vi "Projectile_Range.vi"() -> ()   [LabVIEW 2022 SP3]
panel:
  out "Max Height (m)":dbl
  out "Max Range (m)":dbl
  out "Waveform Graph":dbl[](graph)
  in  "Launch Speed (m/s)":dbl format="%#_13g"
  in  "Launch Angle (deg)":dbl format="%#_13g"
  # "Projectile_Range:\nEnter a value for launch angle and launch speed.\nThe plot will then populate to show the trajectory of the projectile."
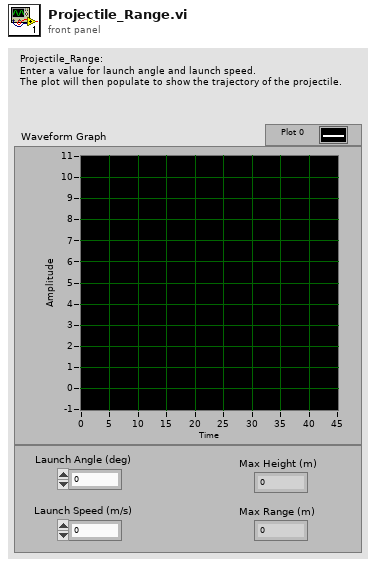
[diagram p1: front panel]
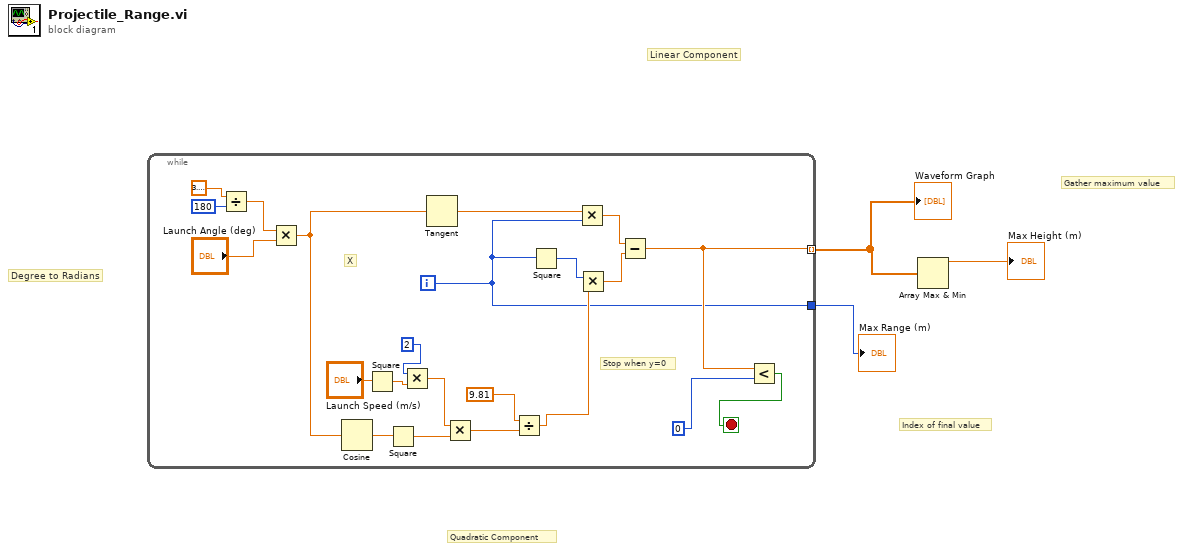
[diagram p0: block diagram]
diagram:
  # "Index of final value"
  # "Gather maximum value"
  # "Quadratic Component"
  # "Linear Component"
  # "Degree to Radians"
  n1 = while {
    tunnel: [w5] -> w3 mode=indexing
    tunnel: [w4] -> w1
    i -> [w4]
    stop <- w6 stop-if-true
    # "Stop when y=0"
    # "X"
    n2 = Divide(x=3.141592653589793, y=180) -> (x/y=w23:dbl)
    n3 = Multiply(x=w23, y="Launch Angle (deg)") -> (x*y=w21:dbl)
    n4 = Cosine(x=w21) -> (cos(x)=w20:dbl)
    n5 = Square(x="Launch Speed (m/s)") -> (x^2=w18:dbl)
    n6 = Square(x=w20) -> (x^2=w16:dbl)
    n7 = Multiply(x=2, y=w18) -> (x*y=w15:dbl)
    n8 = Tangent(1:w21) -> (0:w12:dbl)
    n9 = Multiply(x=w15, y=w16) -> (x*y=w14:dbl)
    n10 = Divide(x=9.81, y=w14) -> (x/y=w11:dbl)
    n11 = Square(x=w4) -> (x^2=w8:i32)
    n12 = Multiply(x=w12, y=w4) -> (x*y=w10:dbl)
    n13 = Multiply(x=w8, y=w11) -> (x*y=w9:dbl)
    n14 = Subtract(x=w10, y=w9) -> (x-y=w5:dbl)
    n15 = Less?(x=w5, y=0) -> (x < y?=w6:bool)
  }
  "Waveform Graph" <- w3
  "Max Range (m)" <- w1
  n16 = Array Max & Min(array=w3) -> (max value=→"Max Height (m)":dbl)  [unwired: 3 out]
